vi "Resolve-action.vi"(8 "error in (no error)":errorcluster, 11 "Message":refnum<class "Message.lvclass">) -> (0 "error out":errorcluster, 2 "Action":T1=enum."Load settings", 3 "Message dup":refnum<class "Message.lvclass">)   [LabVIEW 2013, in "Client.lvlib" / "Client.lvclass"]
uses:
  Client.lvclass
  Messages/Sources/Message.lvclass
  Supported-actions.ctl
  Messages/Sources/Action/Action.lvclass
  Messages/Sources/Action/Action.lvclass/Action.ctl
  Custom-errors.ctl
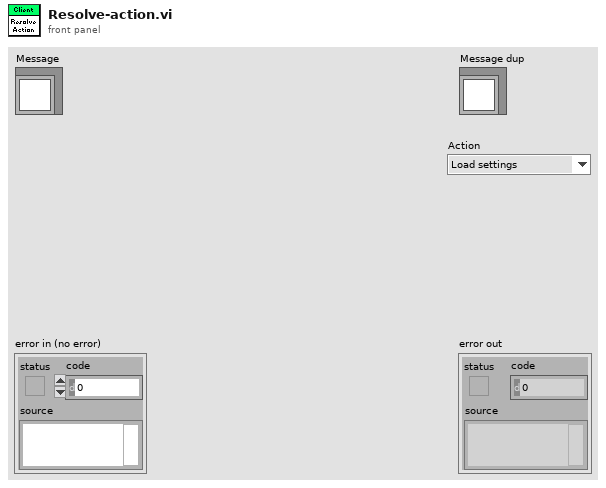
[diagram p1: front panel]
types:
  T1 = typedef "Client.lvlib/Client.lvclass/Supported-actions.ctl" = enum16{"Idle", "Initialize", "Load settings", "Load file", "Ready", "Start", "Pause", "Stop", "Repeat", "Reset", "Exit"}
  T2 = typedef "Client.lvlib/Client.lvclass/Custom-errors.ctl" = enum16{"No error", "Command not recognized", "Invalid input", "Timeout", "Not implemented", "Unsupported message", "Unsupported client", "Unsupported action"}
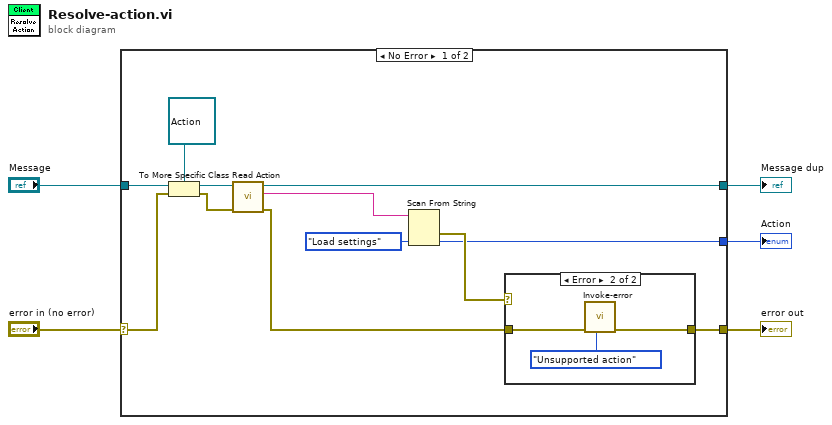
[diagram p0: block diagram]
diagram:
  n1 = case shown="No Error" "error in (no error)" {
    selector: "error in (no error)" -> [w9 w23]
    tunnel: [w15 w23] -> w4
    tunnel: "Message" -> [w10 w22]
    tunnel: [w8 w22] -> w2
    tunnel: [w14 _] -> w1
    frame No Error {
      n2 = To More Specific Class(target class=refnum<class "Action.lvclass"> refnum ("Messages.lvlib:Action.lvclass"), reference=w10, error in=w9) -> (specific class reference=w12:refnum<class "Action.lvclass">, error out=w11:errorcluster)
      n3 = call "Read Action.vi"("error in (no error)"=w11, "Action in"=w12) -> ("error out"=w6:errorcluster, "Action"=w7:string, "Action out"=w8:refnum<class "Action.lvclass">)  [unwired: 7 in]
      n4 = Scan From String(input string=w7, default 1=Supported-actions."Load settings" ("Type")) -> (error out=w16:errorcluster, output 1=w14:T1)  [unwired: 3 in, 2 out]
      n5 = case shown="Error" w16 {
        tunnel: w6 -> [w18 w21]
        tunnel: [w18 w20] -> w15
        frame No Error {
        }
        frame Error {
          n6 = call "Invoke-error.vi"("Error"=Custom-errors."Unsupported action", "error in (no error)"=w21) -> ("error out"=w20:errorcluster)  [unwired: 9 in]
        }
      }
    }
    frame Error {
    }
  }
  "error out" <- w4
  "Message dup" <- w2
  "Action" <- w1
